vi "Processing.vi"(0 "Optional Rectangle":i32[](array[numeric])=[300, 100, 1800, 2050], 1 "Input path":path, 2 "Bj":T1, 5 "BWimag":T1(plugin-control), 7 "Range":cluster{"Lower value":sgl, "Upper value":sgl}={"Lower value"=90.0, "Upper value"=255.0}, 9 "ERthreshold":sgl=-0.1, 11 "Removeareathreshold":i32=2000, 12 "EGthreshold":sgl=0.06, 13 "error in (no error)":errorcluster, 14 "total_RGB":i32) -> (4 "GPAR":dbl, 6 "Bwimag":T1(plugin-control), 10 "original imag":T1(plugin-control))   [LabVIEW 2015]
uses:
  <vilib>/vision/Image Controls.llb/IMAQ Image.ctl
  <vilib>/vision/NI_Vision_Development_Module.lvlib
  Realse/imFillRemove.dll
  remove_blue_pot.dll
  Realse/binarization.dll
panel:
  out "Bwimag 2":T1(plugin-control)
  out "HSL分割结果 2":T1(plugin-control)
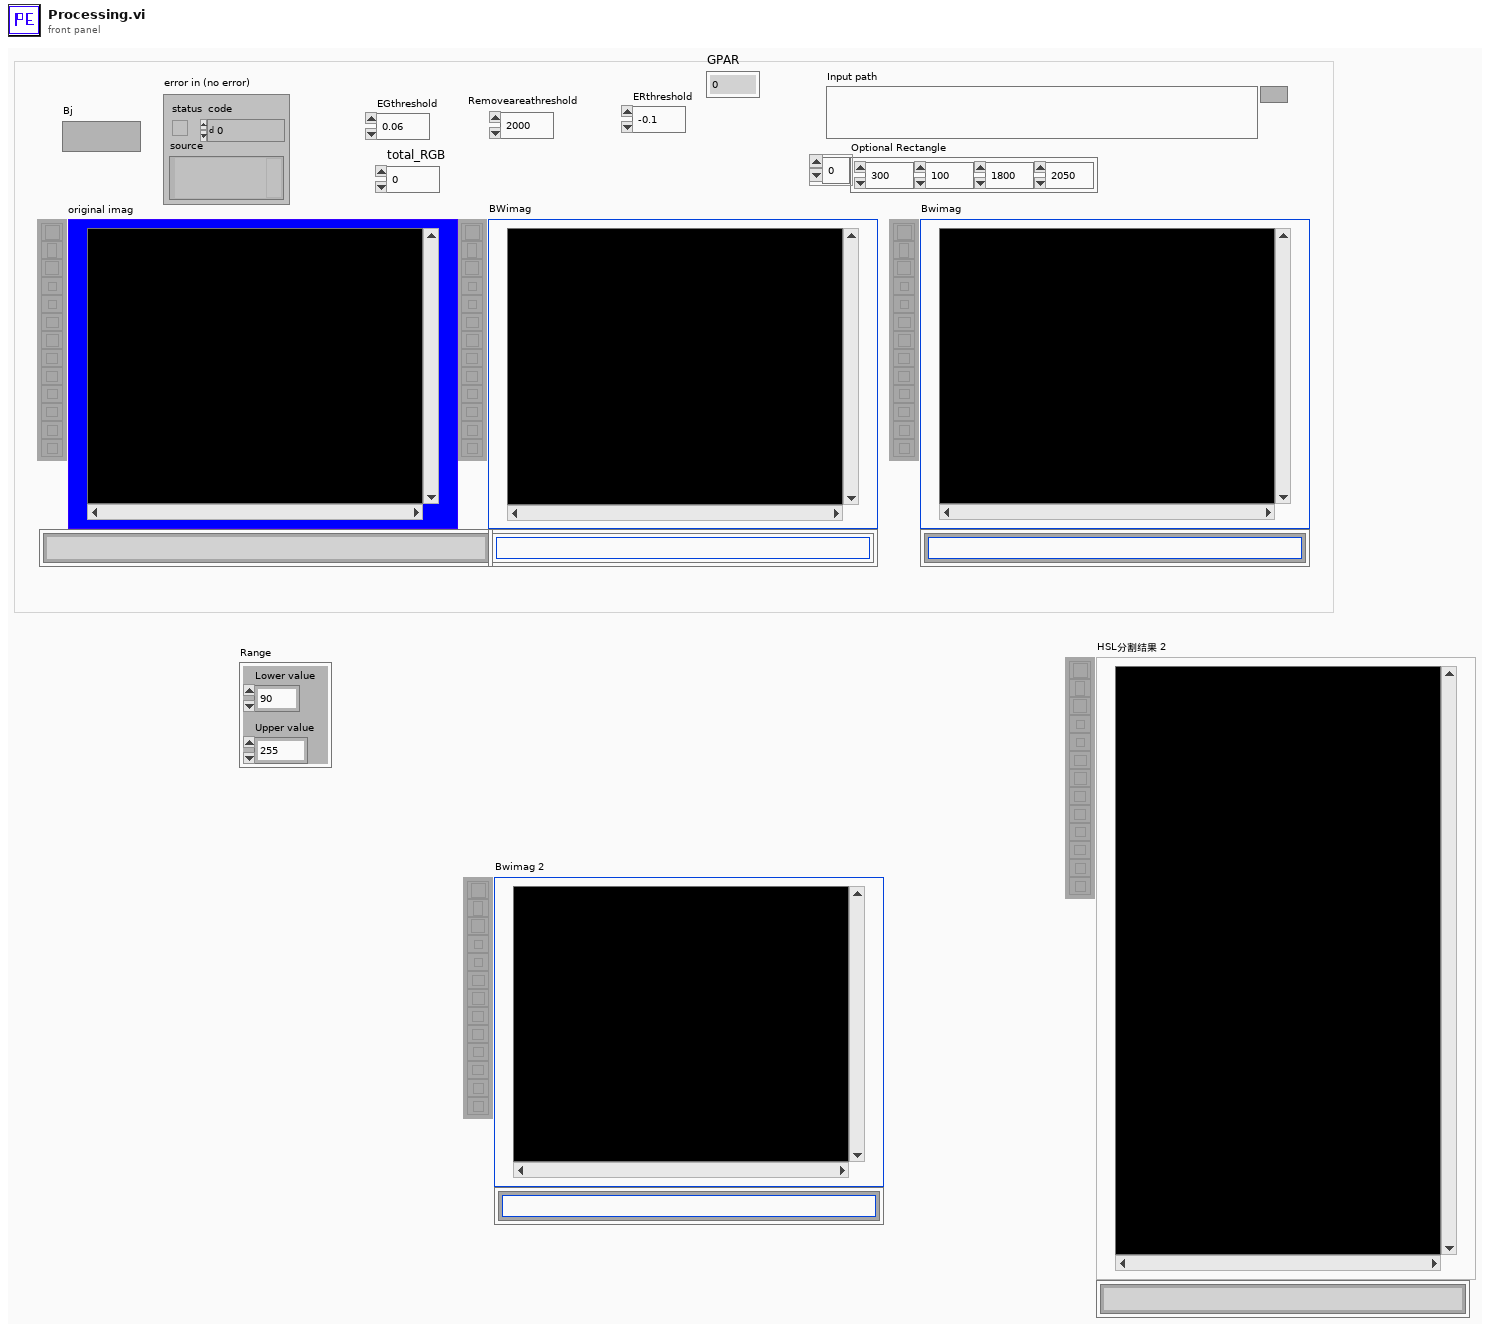
[diagram p1: front panel]
types:
  T1 = typedef "IMAQ Image.ctl" = refnum<image>
  T2 = typedef "Image Type" = u32
  T3 = cluster{"New Image":T1, "New Image":T1, "New Image":T1, "New Image":T1}
  T4 = typedef "Particle Parameters" = i32
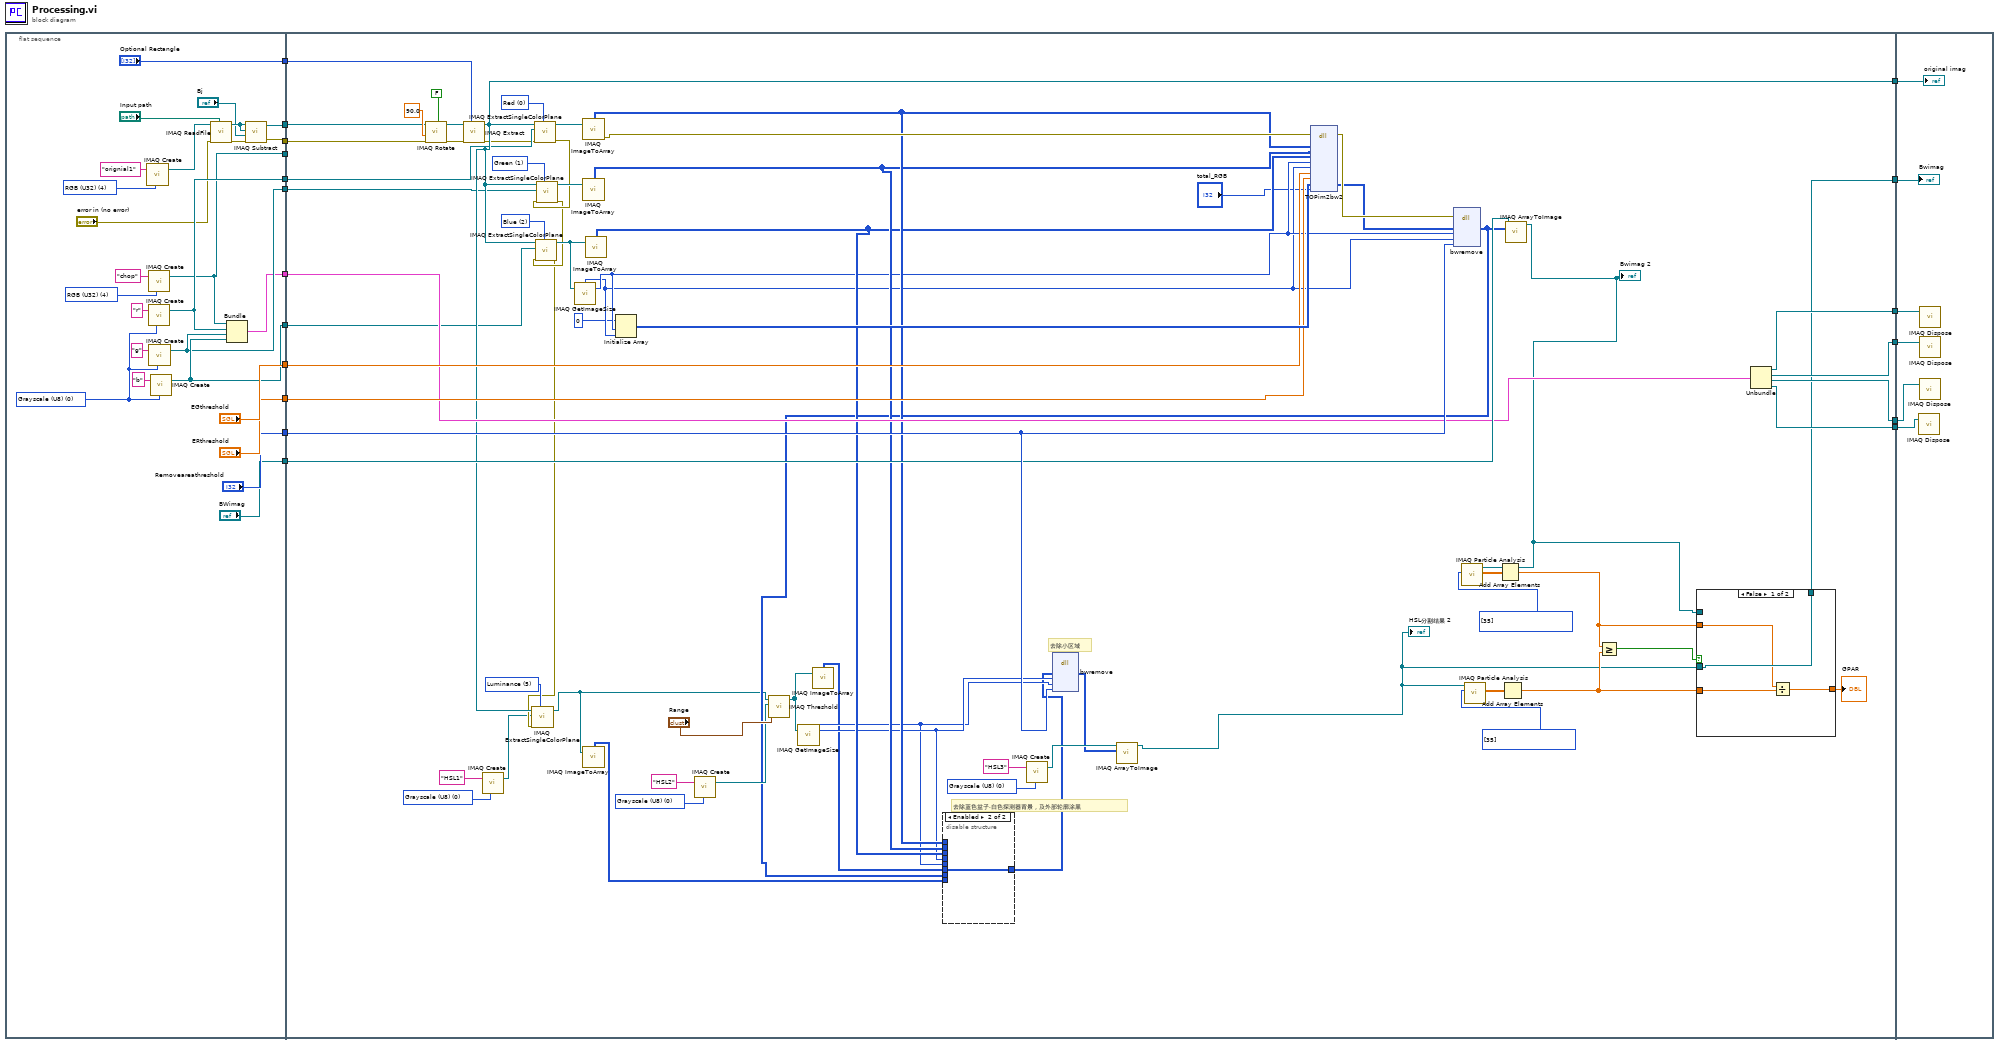
[diagram p0: block diagram]
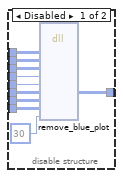
[diagram p2: hidden frame]
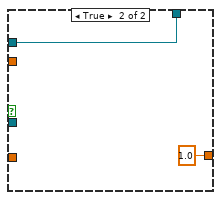
[diagram p3: hidden frame]
diagram:
  n1 = flat-sequence {
    tunnel: [w21] -> w18
    tunnel: [w20] -> w17
    tunnel: [w30] -> w16
    tunnel: ["Optional Rectangle"] -> w15
    tunnel: [w31] -> w14
    tunnel: [w32] -> w13
    tunnel: [w33] -> w12
    tunnel: ["EGthreshold"] -> w11
    tunnel: ["ERthreshold"] -> w10
    tunnel: ["Removeareathreshold"] -> w9
    tunnel: ["BWimag"] -> w8
    tunnel: [w29] -> w6
    tunnel: [w98] -> w7
    tunnel: [w108] -> w5
    tunnel: [w107] -> w4
    tunnel: [w106] -> w3
    tunnel: [w105] -> w2
    tunnel: [w104] -> w1
    tunnel: w6 -> [w109]
    tunnel: w8 -> [w110]
    tunnel: w9 -> [w113]
    tunnel: w10 -> [w114]
    tunnel: w11 -> [w115]
    tunnel: w12 -> [w84]
    tunnel: w13 -> [w85]
    tunnel: w14 -> [w86]
    tunnel: w15 -> [w90]
    tunnel: w16 -> [_]
    tunnel: w17 -> [w78]
    tunnel: w18 -> [w79]
    tunnel: w7 -> [w139]
    tunnel: w5 -> [w138]
    tunnel: w4 -> [w137]
    tunnel: w3 -> [w136]
    tunnel: w2 -> [w135]
    tunnel: w1 -> [w134]
    frame #0 {
      w28 = T2 4 items=["Grayscale (U8)", "Grayscale (I16)", "Grayscale (SGL)", "Complex (CSG)", "RGB (U32)", "HSL (U32)", "RGB (U64)", "Grayscale (U16)"] ("Image Type")
      w39 = T2 4 items=["Grayscale (U8)", "Grayscale (I16)", "Grayscale (SGL)", "Complex (CSG)", "RGB (U32)", "HSL (U32)", "RGB (U64)", "Grayscale (U16)"] ("Image Type")
      w44 = T2 0 items=["Grayscale (U8)", "Grayscale (I16)", "Grayscale (SGL)", "Complex (CSG)", "RGB (U32)", "HSL (U32)", "RGB (U64)", "Grayscale (U16)"] ("Image Type")
      n2 = call "IMAQ Create"("Image Name"="orignial1", "Image Type"=w28) -> ("New Image"=w25:T1)  [unwired: 2 in, 2 out]
      n3 = call "IMAQ Create"("Image Name"="chop", "Image Type"=w39) -> ("New Image"=w30:T1)  [unwired: 2 in, 2 out]
      n4 = call "IMAQ Create"("Image Name"="r", "Image Type"=w44) -> ("New Image"=w31:T1)  [unwired: 2 in, 2 out]
      n5 = call "IMAQ Create"("Image Name"="g", "Image Type"=w44) -> ("New Image"=w32:T1)  [unwired: 2 in, 2 out]
      n6 = call "IMAQ Create"("Image Name"="b", "Image Type"=w44) -> ("New Image"=w33:T1)  [unwired: 2 in, 2 out]
      n7 = call "IMAQ ReadFile"("File Path"="Input path", "error in (no error)"="error in (no error)", "Image"=w25) -> ("error out"=w24:errorcluster, "Image Out"=w23:T1)  [unwired: 2 in, 5 out]
      n8 = Bundle("New Image"=w30, "New Image"=w31, "New Image"=w32, "New Image"=w33) -> (w29:T3)  [unwired: 1 out]
      n9 = call "IMAQ Subtract"("Image Src A"=w23, "Image Dst"=w23, "Image Src B"="Bj", "error in (no error)"=w24) -> ("Image Dst Out"=w21:T1, "error out"=w20:errorcluster)  [unwired: 1 in, 2 out]
    }
    frame #1 {
      w62 = T2 0 items=["Grayscale (U8)", "Grayscale (I16)", "Grayscale (SGL)", "Complex (CSG)", "RGB (U32)", "HSL (U32)", "RGB (U64)", "Grayscale (U16)"] ("Image Type")
      w64 = T2 0 items=["Grayscale (U8)", "Grayscale (I16)", "Grayscale (SGL)", "Complex (CSG)", "RGB (U32)", "HSL (U32)", "RGB (U64)", "Grayscale (U16)"] ("Image Type")
      w73 = T2 0 items=["Grayscale (U8)", "Grayscale (I16)", "Grayscale (SGL)", "Complex (CSG)", "RGB (U32)", "HSL (U32)", "RGB (U64)", "Grayscale (U16)"] ("Image Type")
      w74 = 5 items=["Red", "Green", "Blue", "Hue", "Saturation", "Luminance", "Value", "Intensity"] ("Color Plane")
      w87 = 2 items=["Red", "Green", "Blue", "Hue", "Saturation", "Luminance", "Value", "Intensity"] ("Color Plane")
      w88 = 1 items=["Red", "Green", "Blue", "Hue", "Saturation", "Luminance", "Value", "Intensity"] ("Color Plane")
      w89 = 0 items=["Red", "Green", "Blue", "Hue", "Saturation", "Luminance", "Value", "Intensity"] ("Color Plane")
      w100 = T4[] [35] items=["Center of Mass X", "Center of Mass Y", "First Pixel X", "First Pixel Y", "Bounding Rect Left", "Bounding Rect Top", "Bounding Rect Right", "Bounding Rect Bottom", "Max Feret Diameter Start X", "Max Feret Diameter Start Y", "Max Feret Diameter End X", "Max Feret Diameter End Y", "Max Horiz. Segment Length Left", "Max Horiz. Segment Length Right", "Max Horiz. Segment Length Row", "-", "Bounding Rect Width", "Bounding Rect Height", "Bounding Rect Diagonal", "Perimeter", "Convex Hull Perimeter", "Holes' Perimeter", "Max Feret Diameter", "Equivalent Ellipse Major Axis", "Equivalent Ellipse Minor Axis", "Equivalent Ellipse Minor Axis (Feret)", "Equivalent Rect Long Side", "Equivalent Rect Short Side", "Equivalent Rect Diagonal", "Equivalent Rect Short Side (Feret)", "Average Horiz. Segment Length", "Average Vert. Segment Length", "Hydraulic Radius", "Waddel Disk Diameter", "-", "Area", "Holes' Area", "Particle & Holes' Area", "Convex Hull Area", "Image Area", "-", "Number of Holes", "Number of Horiz. Segments", "Number of Vert. Segments", "-", "Orientation", "Max Feret Diameter Orientation", "-", "% Area/Image Area", "% Area/(Particle & Holes' Area)", "Ratio of Equivalent Ellipse Axes", "Ratio of Equivalent Rect Sides", "-", "Elongation Factor", "Compactness Factor", "Heywood Circularity Factor", "Type Factor", "-", "Sum X", "Sum Y", "Sum XX", "Sum XY", "Sum YY", "Sum XXX", "Sum XXY", "Sum XYY", "Sum YYY", "-", "Moment of Inertia XX", "Moment of Inertia XY", "Moment of Inertia YY", "Moment of Inertia XXX", "Moment of Inertia XXY", "Moment of Inertia XYY", "Moment of Inertia YYY", "Norm. Moment of Inertia XX", "Norm. Moment of Inertia XY", "Norm. Moment of Inertia YY", "Norm. Moment of Inertia XXX", "Norm. Moment of Inertia XXY", "Norm. Moment of Inertia XYY", "Norm. Moment of Inertia YYY", "Hu Moment 1", "Hu Moment 2", "Hu Moment 3", "Hu Moment 4", "Hu Moment 5", "Hu Moment 6", "Hu Moment 7"] ("Pixel Measurements")
      w103 = T4[] [35] items=["Center of Mass X", "Center of Mass Y", "First Pixel X", "First Pixel Y", "Bounding Rect Left", "Bounding Rect Top", "Bounding Rect Right", "Bounding Rect Bottom", "Max Feret Diameter Start X", "Max Feret Diameter Start Y", "Max Feret Diameter End X", "Max Feret Diameter End Y", "Max Horiz. Segment Length Left", "Max Horiz. Segment Length Right", "Max Horiz. Segment Length Row", "-", "Bounding Rect Width", "Bounding Rect Height", "Bounding Rect Diagonal", "Perimeter", "Convex Hull Perimeter", "Holes' Perimeter", "Max Feret Diameter", "Equivalent Ellipse Major Axis", "Equivalent Ellipse Minor Axis", "Equivalent Ellipse Minor Axis (Feret)", "Equivalent Rect Long Side", "Equivalent Rect Short Side", "Equivalent Rect Diagonal", "Equivalent Rect Short Side (Feret)", "Average Horiz. Segment Length", "Average Vert. Segment Length", "Hydraulic Radius", "Waddel Disk Diameter", "-", "Area", "Holes' Area", "Particle & Holes' Area", "Convex Hull Area", "Image Area", "-", "Number of Holes", "Number of Horiz. Segments", "Number of Vert. Segments", "-", "Orientation", "Max Feret Diameter Orientation", "-", "% Area/Image Area", "% Area/(Particle & Holes' Area)", "Ratio of Equivalent Ellipse Axes", "Ratio of Equivalent Rect Sides", "-", "Elongation Factor", "Compactness Factor", "Heywood Circularity Factor", "Type Factor", "-", "Sum X", "Sum Y", "Sum XX", "Sum XY", "Sum YY", "Sum XXX", "Sum XXY", "Sum XYY", "Sum YYY", "-", "Moment of Inertia XX", "Moment of Inertia XY", "Moment of Inertia YY", "Moment of Inertia XXX", "Moment of Inertia XXY", "Moment of Inertia XYY", "Moment of Inertia YYY", "Norm. Moment of Inertia XX", "Norm. Moment of Inertia XY", "Norm. Moment of Inertia YY", "Norm. Moment of Inertia XXX", "Norm. Moment of Inertia XXY", "Norm. Moment of Inertia XYY", "Norm. Moment of Inertia YYY", "Hu Moment 1", "Hu Moment 2", "Hu Moment 3", "Hu Moment 4", "Hu Moment 5", "Hu Moment 6", "Hu Moment 7"] ("Pixel Measurements")
      # "去除蓝色盆子,白色探测器背景，及外部轮廓涂黑"
      # "去除小区域"
      n10 = call "IMAQ Rotate"("Maintain Size"=FALSE, "error in (no error)"=w78, "Angle (degrees)"=sgl 90.0, "Image Src"=w79) -> ("error out"=w70:errorcluster, "Image Dst Out"=w76:T1)  [unwired: 4 in, 2 out]
      n11 = call "IMAQ Extract"("Optional Rectangle"=w90, "error in (no error)"=w70, "Image Src"=w76) -> ("error out"=w69:errorcluster, "Image Dst Out"=w104:T1)  [unwired: 3 in, 4 out]
      n12 = call "IMAQ Create"("Image Name"="HSL1", "Image Type"=w64) -> ("New Image"=w63:T1)  [unwired: 2 in, 2 out]
      n13 = call "IMAQ ExtractSingleColorPlane"("Color Plane"=w89, "error in (no error)"=w69, "Image Dst"=w86, "Image Src"=w104) -> ("error out"=w68:errorcluster, "Image Dst Out"=w83:T1)  [unwired: 6 out]
      n14 = call "IMAQ ExtractSingleColorPlane"("Color Plane"=w88, "error in (no error)"=w68, "Image Dst"=w85, "Image Src"=w104) -> ("error out"=w67:errorcluster, "Image Dst Out"=w82:T1)  [unwired: 6 out]
      n15 = call "IMAQ ExtractSingleColorPlane"("Color Plane"=w87, "error in (no error)"=w67, "Image Dst"=w84, "Image Src"=w104) -> ("error out"=w66:errorcluster, "Image Dst Out"=w81:T1)  [unwired: 6 out]
      n16 = call "IMAQ ExtractSingleColorPlane"("Color Plane"=w74, "error in (no error)"=w66, "Image Dst"=w63, "Image Src"=w104) -> ("Image Dst Out"=w49:T1)  [unwired: 7 out]
      n17 = call "IMAQ GetImageSize"("Image"=w81) -> ("Y Resolution"=w94:i32, "X Resolution"=w93:i32)  [unwired: 1 in, 3 out]
      n18 = call "IMAQ ImageToArray"("Image"=w83) -> ("error out"=w111:errorcluster, "Image Pixels (U8)"=w97:u8[][])  [unwired: 2 in, 4 out]
      n19 = call "IMAQ ImageToArray"("Image"=w82) -> ("Image Pixels (U8)"=w96:u8[][])  [unwired: 2 in, 5 out]
      n20 = call "IMAQ ImageToArray"("Image"=w49) -> ("Image Pixels (U8)"=w48:u8[][])  [unwired: 2 in, 5 out]
      n21 = call "IMAQ ImageToArray"("Image"=w81) -> ("Image Pixels (U8)"=w95:u8[][])  [unwired: 2 in, 5 out]
      n22 = Initialize Array(u8 0 ("element"), w94, w93) -> (w116:u8[][])
      n23 = call "IMAQ Create"("Image Name"="HSL2", "Image Type"=w62) -> ("New Image"=w60:T1)  [unwired: 2 in, 2 out]
      n24 = call "IMAQ Threshold"("Range"="Range", "Image Dst"=w60, "Image Src"=w49) -> ("Image Dst Out"=w50:T1)  [unwired: 3 in, 5 out]
      n25 = call "IMAQ GetImageSize"("Image"=w50) -> ("Y Resolution"=w58:i32, "X Resolution"=w57:i32)  [unwired: 1 in, 3 out]
      n26 = call "IMAQ ImageToArray"("Image"=w50) -> ("Image Pixels (U8)"=w56:u8[][])  [unwired: 2 in, 5 out]
      n27 = call "IMAQ Create"("Image Name"="HSL3", "Image Type"=w73) -> ("New Image"=w71:T1)  [unwired: 2 in, 2 out]
      n28 = dll-call lib="PTH2iabs E文章投稿&51. 代明球老师-玉米胁迫实验\tRGB程序maizeRealsebinarization.dll" fn="TOPim2bw2"(error in=w111, "R"=w97, "G"=w96, "B"=w95, "row"=w94, "col"=w93, "EGthreshold"=w115, "ERthreshold"=w114, "bw"=w116, "total_RGB"="total_RGB") -> (error out=w112:errorcluster, "bw"=w45:u8[][])  [unwired: 7 in, 5 out]
      n29 = dll-call lib="PTH2iabs E文章投稿&51. 代明球老师-玉米胁迫实验\tRGB程序maizeRealseimFillRemove.dll" fn="bwremove"(error in=w112, "bw"=w45, "row"=w94, "col"=w93, "areathreshold"=w113) -> ("bw"=w54:u8[][])  [unwired: 5 in, 3 out]
      n30 = disable-structure shown="Enabled" {
        disable-tunnel: w97 -> [w126 _]
        disable-tunnel: w96 -> [w125 _]
        disable-tunnel: w95 -> [w124 _]
        disable-tunnel: w58 -> [w123 _]
        disable-tunnel: w57 -> [w122 _]
        disable-tunnel: w56 -> [w121 w127]
        disable-tunnel: [w120 w127] -> w55
        disable-tunnel: w54 -> [w119 _]
        disable-tunnel: w48 -> [w118 _]
        frame Disabled {
          n31 = dll-call lib="PTH2dabs E文章投稿&51. 代明球老师-玉米胁迫实验\tRGB程序maizeremove_blue_pot.dll" fn="remove_blue_plot"("R"=w126, "G"=w125, "B"=w124, "row"=w123, "col"=w122, "bw"=w121, "bw_EG"=w119, "bw_gray_L"=w118, "L_threshold"=u8 30) -> ("bw"=w120:u8[][])  [unwired: 10 in, 4 out]
        }
        frame Enabled {
        }
      }
      n32 = dll-call lib="PTH2iabs E文章投稿&51. 代明球老师-玉米胁迫实验\tRGB程序maizeRealseimFillRemove.dll" fn="bwremove"("bw"=w55, "row"=w58, "col"=w57, "areathreshold"=w113) -> ("bw"=w59:u8[][])  [unwired: 6 in, 3 out]
      n33 = call "IMAQ ArrayToImage"("Image Pixels (U8)"=w59, "Image"=w71) -> ("Image Out"=w46:T1)  [unwired: 4 in, 5 out]
      "HSL分割结果 2" <- w46
      n34 = call "IMAQ Particle Analysis"("Pixel Measurements"=w103, "Image"=w46) -> ("Particle Measurements (Pixels)"=w102:dbl[][])  [unwired: 3 in, 6 out]
      n35 = Add Array Elements(numeric array=w102) -> (sum=w52:dbl)
      n36 = call "IMAQ ArrayToImage"("Image Pixels (U8)"=w54, "Image"=w110) -> ("Image Out"=w92:T1)  [unwired: 4 in, 5 out]
      "Bwimag 2" <- w92
      n37 = call "IMAQ Particle Analysis"("Pixel Measurements"=w100, "Image"=w92) -> ("Particle Measurements (Pixels)"=w101:dbl[][])  [unwired: 3 in, 6 out]
      n38 = Add Array Elements(numeric array=w101) -> (sum=w53:dbl)
      n39 = Greater Or Equal?(x=w53, y=w52) -> (x >= y?=w99:bool)
      n40 = case shown="False" w99 {
        tunnel: w92 -> [_ w133]
        tunnel: [w131 w133] -> w98
        tunnel: w46 -> [w131 _]
        tunnel: w53 -> [w130 _]
        tunnel: w52 -> [w129 _]
        tunnel: [w128 1.0] -> w51
        frame False {
          n41 = Divide(x=w130, y=w129) -> (x/y=w128:dbl)
        }
        frame True {
        }
      }
      "GPAR" <- w51
      n42 = Unbundle(w109) -> ("New Image"=w108:T1, "New Image"=w107:T1, "New Image"=w106:T1, "New Image"=w105:T1)
    }
    frame #2 {
      n43 = call "IMAQ Dispose"("Image"=w135) -> ()  [unwired: 2 in, 4 out]
      n44 = call "IMAQ Dispose"("Image"=w136) -> ()  [unwired: 2 in, 4 out]
      n45 = call "IMAQ Dispose"("Image"=w138) -> ()  [unwired: 2 in, 4 out]
      n46 = call "IMAQ Dispose"("Image"=w137) -> ()  [unwired: 2 in, 4 out]
      "Bwimag" <- w139
      "original imag" <- w134
    }
  }
